vi "Periodic Random Noise Waveform.vi"(6 "sampling info":cluster{"Fs":dbl, "#s":dbl}={"Fs"=1000.0, "#s"=1000.0} {"Fs" format="%.2p"}, 7 "reset signal":bool, 8 "error in (no error)":errorcluster, 10 "seed":i32=-1, 11 "spectral amplitude":dbl=1.0 format="%.2p") -> (0 "error out":errorcluster, 3 "signal out":waveform(dbl))   [LabVIEW 2020, in "NI_MABase.lvlib"]
doc: "Generates a waveform containing periodic random noise (PRN)."
uses:
  NI_MABase.lvlib
  NI_AALBase.lvlib
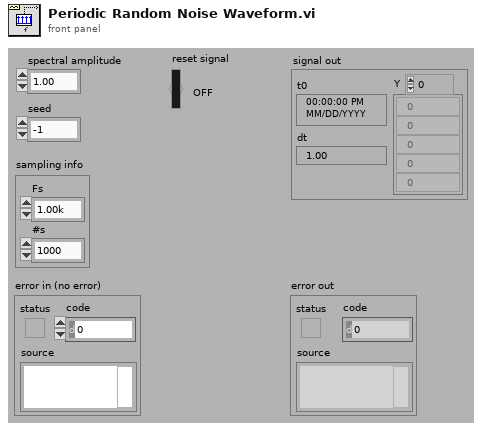
[diagram p1: front panel]
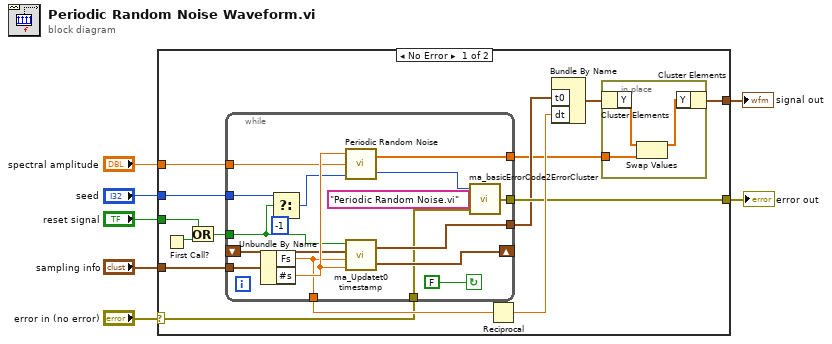
[diagram p0: block diagram]
diagram:
  n1 = case shown="No Error" "error in (no error)" {
    selector: "error in (no error)" -> [w15 w42]
    tunnel: [w20 w42] -> w7
    tunnel: "sampling info" -> [w19 _]
    tunnel: "seed" -> [w17 _]
    tunnel: "spectral amplitude" -> [w16 _]
    tunnel: [w9 _] -> w2
    tunnel: "reset signal" -> [w11 _]
    frame No Error {
      n2 = First Call?() -> (First Call?: T/F=w13:bool)
      n3 = Or(x=w11, y=w13) -> (x .or. y?=w12:bool)
      n4 = while {
        tunnel: w15 -> [w29]
        tunnel: w16 -> [w30]
        tunnel: w17 -> [w27]
        tunnel: w12 -> [w28]
        tunnel: [w33] -> w18
        tunnel: w19 -> [w34]
        tunnel: [w36] -> w8
        tunnel: [w37] -> w14
        shift-left: _ -> [w39]
        shift-right: [w38] -> _
        tunnel: [w40] -> w20
        stop <- FALSE continue-if-true
        n5 = Unbundle By Name(w34) -> ("Fs"=w33:dbl, "#s"=w41:dbl)
        n6 = Select(t=w27, s=w28, f=-1) -> (s? t:f=w26:i32)
        n7 = call "Periodic Random Noise.vi"("seed"=w26, "spectral amplitude"=w30, "samples"=w41) -> ("error"=w32:i32, "periodic random noise"=w36:dbl[])
        n8 = call "ma_Updatet0 timestamp.vi"("samples"=w41, "sampling rate (S/s)"=w33, "tf previous"=w39, "Reset Generation"=w28) -> ("tf new"=w38:timestamp, "t0"=w37:timestamp)
        n9 = call "ma_basicErrorCode2ErrorCluster.vi"("error in (no error)"=w29, "subVI name"="Periodic Random Noise.vi" ("subVI Name"), "Error Code"=w32) -> ("error out"=w40:errorcluster)
      }
      n10 = Reciprocal(x=w18) -> (1/x=w21:dbl)
      n11 = Bundle By Name("t0"=w14, "dt"=w21) -> (w10:waveform(dbl))  [unwired: 1 out]
      n12 = in-place {
        in-place-border: w8 -> [w22]
        n13 = in-place-cluster #1(w10) -> ("Y"=w24:dbl[])
        n14 = Swap Values(12:w24, 14:w22) -> (1:w23:dbl[])  [unwired: 1 in, 1 out]
        n15 = in-place-cluster #1("Y"=w23) -> (w9:waveform(dbl))
      }
    }
    frame Error {
    }
  }
  "error out" <- w7
  "signal out" <- w2
